vi "spots_shape.vi"(6 "Selection and Groups":T1[](array[typedef]), 9 "Spots":T2[](array[typedef]) {"Amplitude Correction" step=0.1; "Line Trapping"."Phase Gradient" step=0.05; "Line Trapping"."Vector"."x" step=1e-06 format="%#_6p"; "Line Trapping"."Vector"."y" step=1e-06 format="%#_6p"; "Line Trapping"."Vector"."z" step=1e-06 format="%#_6p"; "NA Position"."r" step=1e-06; "NA Position"."y" step=1e-06; "NA Position"."x" step=1e-06; "Position"."z" step=1e-06; "Position"."y" step=1e-06; "Position"."x" step=1e-06; "Phase" step=0.7753; "Intensity" step=0.1}) -> (2 "Spot Shape":enum32{"Normal", "Line", "NA", "Mixed"}(ring))   [LabVIEW 2015]
uses:
  spot.ctl
  line_trapping.ctl
  selection_element.ctl
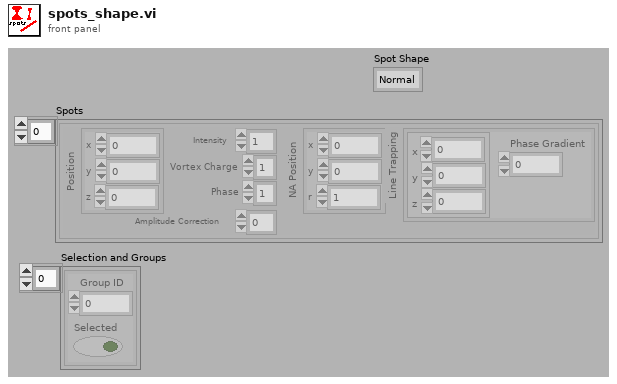
[diagram p1: front panel]
types:
  T1 = typedef "selection_element.ctl" = cluster{"Group ID":i32, "Selected":bool}
  T2 = typedef "spot.ctl" = cluster{"Position":cluster{"x":dbl, "y":dbl, "z":dbl}, "Intensity":dbl, "Vortex Charge":i8, "Phase":dbl, "NA Position":cluster{"x":dbl, "y":dbl, "r":dbl}, "Line Trapping":T3, "Amplitude Correction":dbl}
  T3 = typedef "line_trapping.ctl" = cluster{"Vector":cluster{"x":dbl, "y":dbl, "z":dbl}, "Phase Gradient":dbl}
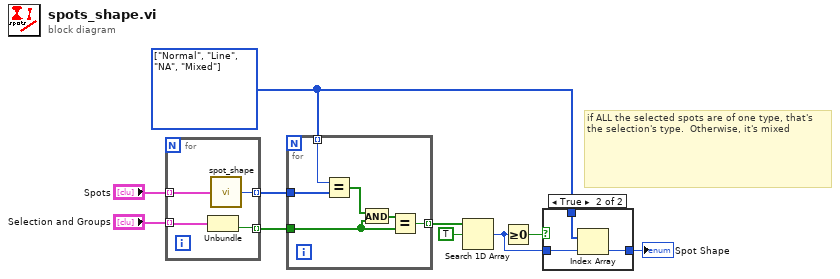
[diagram p0: block diagram]
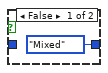
[diagram p2: hidden frame]
diagram:
  w2 = enum32{"Normal", "Line", "NA", "Mixed"}[] [enum."Normal", enum."Line", enum."NA", enum."Mixed"] items=["Normal", "Line", "NA", "Mixed"]
  # "if ALL the selected spots are of one type, that's the selection's type.  Otherwise, it's mixed"
  n1 = for {
    tunnel: "Selection and Groups" -> [w12] mode=indexing
    tunnel: "Spots" -> [w14] mode=indexing
    tunnel: [w13] -> w8 mode=indexing
    tunnel: [w11] -> w7 mode=indexing
    n2 = Unbundle(w12) -> ("Selected"=w11:bool)  [unwired: 1 out]
    n3 = call "spot_shape.vi"("Spot"=w14) -> ("Spot Shape"=w13:enum32{"Normal", "Line", "NA", "Mixed"})
  }
  n4 = for {
    tunnel: w2 -> [w19] mode=indexing
    tunnel: w8 -> [w20]
    tunnel: w7 -> [w16]
    tunnel: [w18] -> w6 mode=indexing
    n5 = Equal?(x=w19, y=w20) -> (x = y?=w15:bool[])
    n6 = And(x=w15, y=w16) -> (x .and. y?=w17:bool[])
    n7 = Equal?(x=w17, y=w16) -> (x = y?=w18:bool)
  }
  n8 = Search 1D Array(1D array=w6, element=TRUE) -> (index of element=w3:i32)  [unwired: 1 in]
  n9 = Greater Or Equal To 0?(x=w3) -> (x >= 0?=w4:bool)
  n10 = case shown="True" w4 {
    tunnel: w3 -> [_ w24]
    tunnel: w2 -> [_ w23]
    tunnel: [enum32{"Normal", "Line", "NA", "Mixed"}."Mixed" ("f") w22] -> w1
    frame False {
    }
    frame True {
      n11 = Index Array(array=w23, index=w24) -> (element=w22:enum32{"Normal", "Line", "NA", "Mixed"})
    }
  }
  "Spot Shape" <- w1
